vi "Declare Dependency.vi"(6 "Shared Resource":bool, 8 "error in (no error)":errorcluster, 9 "Name":string, 10 "Dependency":refnum<class "SMO.lvclass">, 11 "SMO in":refnum<class "SMO.lvclass">) -> (0 "error out":errorcluster, 1 "Unique Name":string, 2 "Dependency out":refnum<class "SMO.lvclass">, 3 "SMO out":refnum<class "SMO.lvclass">)   [LabVIEW 2013, in "SMO.lvclass"]
uses:
  SMO.lvclass
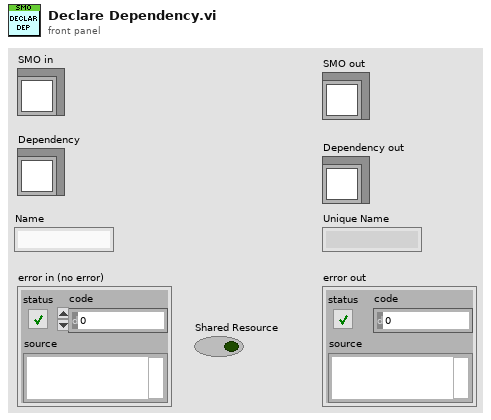
[diagram p1: front panel]
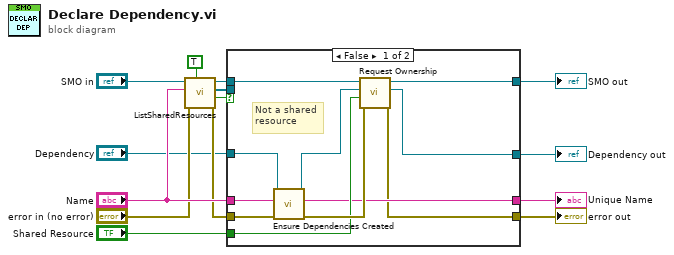
[diagram p0: block diagram]
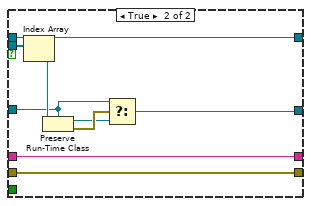
[diagram p2: hidden frame]
diagram:
  n1 = call "ListSharedResources.vi"("exact name? (F: regex)"=TRUE, "error in (no error)"="error in (no error)", "Filter (regex|name)"="Name", "SMO in"="SMO in") -> ("error out"=w11:errorcluster, "resources found?"=w7:bool, "Shared Resources"=w4:refnum<class "SMO.lvclass">[], "SMO out"=w5:refnum<class "SMO.lvclass">)  [unwired: 4 in]
  n2 = case shown="False" w7 {
    tunnel: w4 -> [_ w34]
    tunnel: w5 -> [w24 w33]
    tunnel: [w23 w33] -> w6
    tunnel: [w22 w29] -> w8
    tunnel: "Dependency" -> [w18 w28]
    tunnel: "Name" -> [w25 w26]
    tunnel: w11 -> [w21 w27]
    tunnel: [w15 w27] -> w12
    tunnel: "Shared Resource" -> [w19 _]
    tunnel: [w16 w26] -> w1
    frame False {
      # "Not a shared\nresource"
      n3 = call "Ensure Dependencies Created.vi"("error in (no error)"=w21, "Dependency Name"=w25, "SMO in"=w18) -> ("error out"=w20:errorcluster, "Unique Dependency name"=w16:string, "SMO out"=w17:refnum<class "SMO.lvclass">)  [unwired: 6 in]
      n4 = call "Request Ownership.vi"("error in (no error)"=w20, "Shared Resource"=w19, "Dependency"=w17, "SMO in"=w24) -> ("error out"=w15:errorcluster, "Dependency out"=w22:refnum<class "SMO.lvclass">, "SMO out"=w23:refnum<class "SMO.lvclass">)  [unwired: 5 in]
    }
    frame True {
      n5 = Index Array(array=w34) -> (element=w32:refnum<class "SMO.lvclass">)  [unwired: 1 in]
      n6 = Preserve Run-Time Class(object in=w32, 2:w28) -> (object out=w30:refnum<class "SMO.lvclass">, error out=w31:errorcluster)  [unwired: 1 in]
      n7 = Select(t=w28, s=w31, f=w30) -> (s? t:f=w29:refnum<class "SMO.lvclass">)
    }
  }
  "error out" <- w12
  "Dependency out" <- w8
  "SMO out" <- w6
  "Unique Name" <- w1
